vi "Manual Gear Aim.vi"(9 "Rotate In":dbl, 10 "Y In":dbl, 11 "X Input":dbl) -> (1 "Rotate Out":dbl, 2 "Y Out":dbl, 3 "X Out":dbl)   [LabVIEW 2016]
uses:
  Robot Global Data.vi
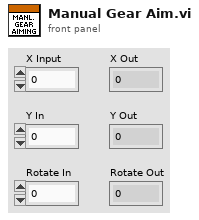
[diagram p1: front panel]
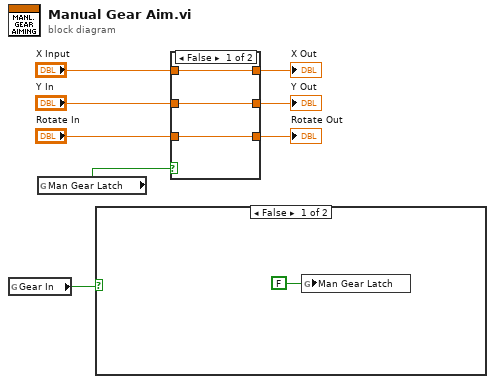
[diagram p0: block diagram]
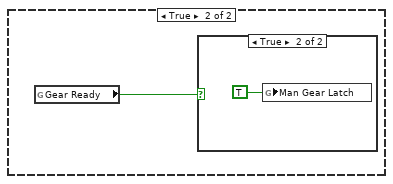
[diagram p2: hidden frame]
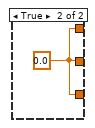
[diagram p4: hidden frame]
diagram:
  n1 = global read "Robot Global Data.vi" "Gear In"() -> (w1:bool)
  n2 = global read "Robot Global Data.vi" "Man Gear Latch"() -> (w2:bool)
  n3 = case shown="False" w1 {
    frame False {
      n4 = global write "Robot Global Data.vi" "Man Gear Latch"(FALSE ("Latch")) -> ()
    }
    frame True {
      n5 = global read "Robot Global Data.vi" "Gear Ready"() -> (w10:bool)
      n6 = case shown="True" w10 {
        frame False {
        }
        frame True {
          n7 = global write "Robot Global Data.vi" "Man Gear Latch"(TRUE ("Latch")) -> ()
        }
      }
    }
  }
  n8 = case shown="False" w2 {
    tunnel: [w14 w15] -> w3
    tunnel: "X Input" -> [w14 _]
    tunnel: [w13 w15] -> w5
    tunnel: "Y In" -> [w13 _]
    tunnel: [w12 w15] -> w7
    tunnel: "Rotate In" -> [w12 _]
    frame False {
    }
    frame True {
      w15 = 0.0
    }
  }
  "Rotate Out" <- w7
  "Y Out" <- w5
  "X Out" <- w3
